vi "calculate next level.vi"(10 "pascal's triangle":dbl[](array[numeric])) -> (2 "next level":dbl[](array[numeric]))   [LabVIEW 2009]
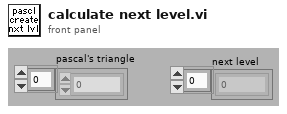
[diagram p1: front panel]
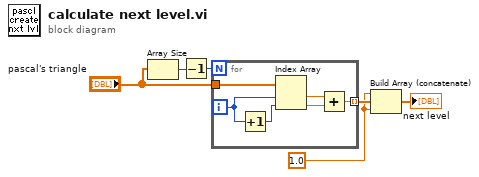
[diagram p0: block diagram]
diagram:
  w1 = 1.0 ("element")
  n1 = Array Size(array="pascal's triangle") -> (size(s)=w6:i32)
  n2 = Decrement(x=w6) -> (x-1=w5:i32)
  n3 = for {
    N: w5 -> [_]
    tunnel: "pascal's triangle" -> [w12]
    tunnel: [w7] -> w3 mode=indexing
    i -> [w11]
    n4 = Increment(x=w11) -> (x+1=w10:i32)
    n5 = Index Array(array=w12, index #1=w11, index #2=w10) -> (element #1=w8:dbl, element #2=w9:dbl)
    n6 = Add(x=w8, y=w9) -> (x+y=w7:dbl)
  }
  n7 = Build Array (concatenate)(w1, w3, w1) -> (→"next level":dbl[])
